vi "Close Transport.vi"(8 "error in (no error)":errorcluster, 11 "EventTransport":refnum<class "EventTransport.lvclass">) -> (0 "error out":errorcluster)   [LabVIEW 2020, in "EventTransport.lvclass"]
doc: "关闭传输"
uses:
  EventTransport.lvclass
  EventTransport.lvclass/EventTransport.ctl
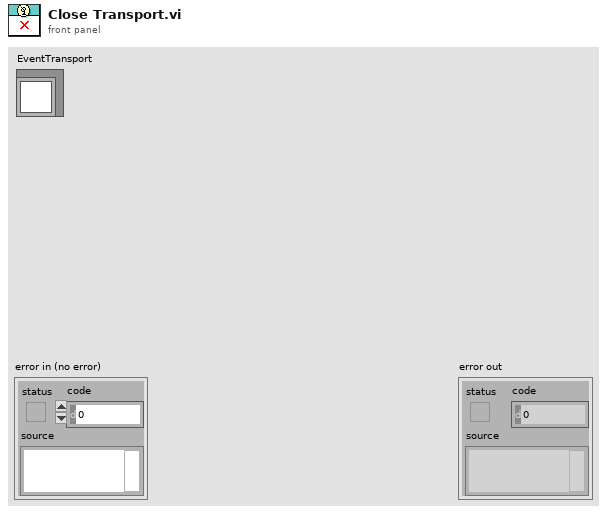
[diagram p1: front panel]
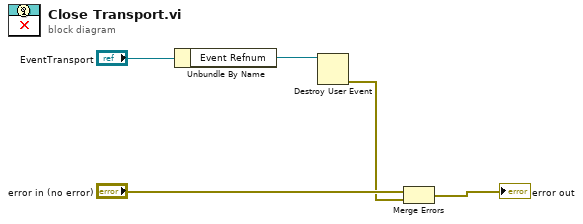
[diagram p0: block diagram]
diagram:
  n1 = Unbundle By Name("EventTransport") -> ("Event Refnum"=w2:refnum<user-event>)
  n2 = Destroy User Event(user event=w2) -> (error out=w1:errorcluster)  [unwired: 1 in]
  n3 = Merge Errors("error in (no error)", w1) -> (→"error out":errorcluster)
